vi "simple pipelines.vi"() -> ()   [LabVIEW 2013]
uses:
  protocol.ctl
  domain.ctl
  TX and RX flags.ctl
  lvnano.lvlib
  nanomsg.dll
panel:
  out "error out":errorcluster
  out "string":string
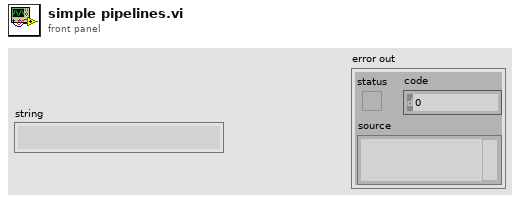
[diagram p1: front panel]
types:
  T1 = typedef "lvnano.lvlib/TX and RX flags.ctl" = i32
  T2 = typedef "lvnano.lvlib/protocol.ctl" = i32
  T3 = typedef "lvnano.lvlib/domain.ctl" = enum16{"Invalid", "AF_SP", "AF_SP_RAW"}
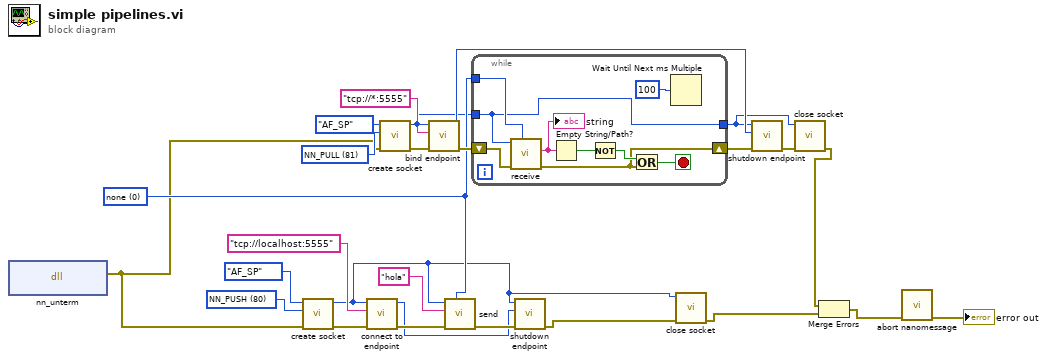
[diagram p0: block diagram]
diagram:
  w14 = T1 0 items=["none", "NN_DONTWAIT"] ("receive flags")
  w21 = T2 80 items=["NN_PUSH"=80, "NN_PULL"=81] ("protocol")
  w24 = T2 81 items=["NN_PUSH"=80, "NN_PULL"=81] ("protocol")
  n1 = dll-call lib="C:/Users/Daniel/Desktop/lvnano/nanomsg.*" fn="nn_unterm"() -> (error out=w2:errorcluster)  [unwired: 4 in, 1 out]
  n2 = call "create socket.vi"("error in"=w2, "protocol"=w21, "domain"=domain."AF_SP") -> ("error out"=w19:errorcluster, "socket"=w11:i32)  [unwired: 7 in]
  n3 = call "connect to endpoint.vi"("error in"=w19, "address"="tcp://localhost:5555" ("addr"), "socket"=w11) -> ("error out"=w17:errorcluster, "endpoint"=w6:i32)  [unwired: 7 in]
  n4 = call "create socket.vi"("error in"=w2, "protocol"=w24, "domain"=domain."AF_SP") -> ("error out"=w26:errorcluster, "socket"=w4:i32)  [unwired: 7 in]
  n5 = call "bind endpoint.vi"("error in"=w26, "address"="tcp://*:5555" ("addr"), "socket"=w4) -> ("error out"=w22:errorcluster, "endpoint"=w5:i32)  [unwired: 7 in]
  n6 = call "send.vi"("flags"=w14, "error in"=w17, "data"="hola" ("String"), "socket"=w11) -> ("error out"=w16:errorcluster)  [unwired: 7 in]
  n7 = while {
    tunnel: w14 -> [w33]
    shift-right: [w28] -> w13
    shift-left: w22 -> [w35]
    tunnel: w4 -> [w27]
    tunnel: [w27] -> w3
    stop <- w30 stop-if-true
    n8 = call "receive.vi"("flags"=w33, "error in"=w35, "socket"=w27) -> ("error out"=w28:errorcluster, "data"=w34:string)  [unwired: 7 in]
    "string" <- w34
    n9 = Empty String/Path?(string/path=w34) -> (empty?=w31:bool)
    n10 = Not(x=w31) -> (.not. x?=w29:bool)
    n11 = Or(x=w29, y=w28) -> (x .or. y?=w30:bool)
    n12 = Wait Until Next ms Multiple(millisecond multiple=u32 100) -> ()  [unwired: 1 out]
  }
  n13 = call "shutdown endpoint.vi"("error in"=w16, "endpoint"=w6, "socket"=w11) -> ("error out"=w10:errorcluster)  [unwired: 8 in]
  n14 = call "close socket.vi"("error in"=w10, "socket"=w11) -> ("error out"=w8:errorcluster)  [unwired: 9 in]
  n15 = call "shutdown endpoint.vi"("error in"=w13, "endpoint"=w5, "socket"=w3) -> ("error out"=w12:errorcluster)  [unwired: 8 in]
  n16 = call "close socket.vi"("error in"=w12, "socket"=w3) -> ("error out"=w9:errorcluster)  [unwired: 9 in]
  n17 = Merge Errors(w9, w8) -> (w7:errorcluster)
  n18 = call "abort nanomessage.vi"("error in"=w7) -> ("error out"=→"error out":errorcluster)  [unwired: 10 in]
